vi "Init_UI_Cluster.vi"(0 "UI_Cluster_In":T1, 3 "error in":errorcluster) -> (7 "UI_Cluster_Out":T1, 10 "error out":errorcluster)   [LabVIEW 2020]
uses:
  Type_Def/UI_Ref_Cluster.ctl
  controls/Car_wash_indicators.ctl
  controls/Wash_options.ctl
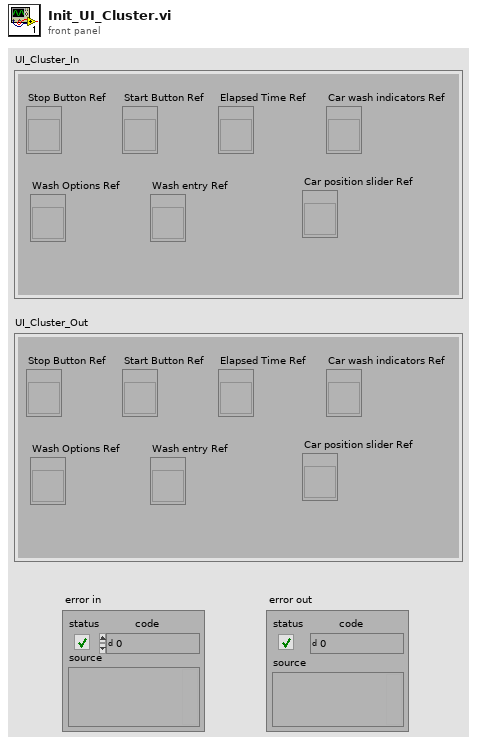
[diagram p1: front panel]
types:
  T1 = typedef "UI_Ref_Cluster.ctl" = cluster{"Stop Button Ref":refnum<vi>, "Start Button Ref":refnum<vi>, "Elapsed Time Ref":refnum<vi>, "Car wash indicators Ref":refnum<vi>, "Wash Options Ref":refnum<vi>, "Wash entry Ref":refnum<vi>, "Car position slider Ref":refnum<vi>}
  T2 = enum8{"Enabled", "Disabled", "Disabled and Grayed Out"}
  T3 = typedef "Wash_options.ctl" = cluster{"Under body wash":bool, "Bug remover":bool, "Pre-soak":bool, "High pressure":bool, "Low pressure":bool, "Spot free Rinse":bool, "Tire Shine Foam":bool, "Air Dry":bool}
  T4 = typedef "Car_wash_indicators.ctl" = cluster{"Under Body Wash":bool, "Bug remover":bool, "Pre-soak":bool, "High pressure Wash":bool, "Low pressure Wax":bool, "Spot free Rinse ":bool, "Tire Shine Foam ":bool, "Air Dry ":bool, "Vehicle Out of Position":bool}
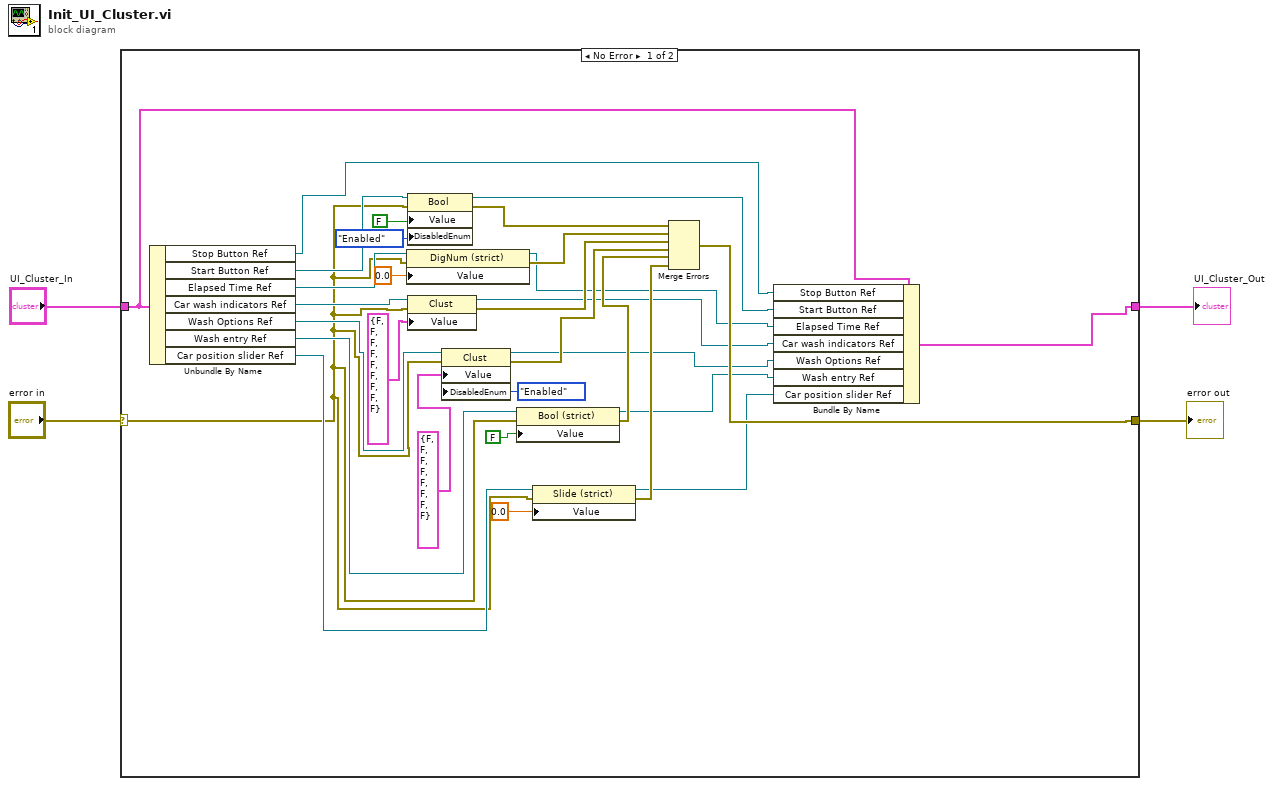
[diagram p0: block diagram]
diagram:
  n1 = case shown="No Error" "error in" {
    selector: "error in" -> [w18 w37]
    tunnel: [w16 w37] -> w3
    tunnel: "UI_Cluster_In" -> [w15 w36]
    tunnel: [w8 w36] -> w1
    frame No Error {
      n2 = Unbundle By Name(w15) -> ("Stop Button Ref"=w7:refnum<vi>, "Start Button Ref"=w35:refnum<vi>, "Elapsed Time Ref"=w32:refnum<vi>, "Car wash indicators Ref"=w29:refnum<vi>, "Wash Options Ref"=w26:refnum<vi>, "Wash entry Ref"=w23:refnum<vi>, "Car position slider Ref"=w22:refnum<vi>)
      n3 = property class="DigNum (strict)"(reference=w32, error in=w18, "Value"=0.0) -> (reference out=w13:refnum<vi>, error out=w30:errorcluster)
      n4 = property class="Bool"(reference=w35, error in=w18, "Value"=FALSE, "DisabledEnum"=T2."Enabled" ("Disabled")) -> (reference out=w14:refnum<vi>, error out=w33:errorcluster)
      n5 = property class="Clust"(reference=w29, error in=w18, "Value"=T4 {"Under Body Wash"=FALSE, "Bug remover"=FALSE, "Pre-soak"=FALSE, "High pressure Wash"=FALSE, "Low pressure Wax"=FALSE, "Spot free Rinse "=FALSE, "Tire Shine Foam "=FALSE, "Air Dry "=FALSE, "Vehicle Out of Position"=FALSE} ("Car wash indicators")) -> (reference out=w12:refnum<vi>, error out=w28:errorcluster)
      n6 = property class="Clust"(reference=w26, error in=w18, "Value"=T3 {"Under body wash"=FALSE, "Bug remover"=FALSE, "Pre-soak"=FALSE, "High pressure"=FALSE, "Low pressure"=FALSE, "Spot free Rinse"=FALSE, "Tire Shine Foam"=FALSE, "Air Dry"=FALSE} ("Wash Options"), "DisabledEnum"=T2."Enabled" ("Disabled")) -> (reference out=w11:refnum<vi>, error out=w24:errorcluster)
      n7 = property class="Bool (strict)"(reference=w23, error in=w18, "Value"=FALSE) -> (reference out=w10:refnum<vi>, error out=w20:errorcluster)
      n8 = property class="Slide (strict)"(reference=w22, error in=w18, "Value"=0.0) -> (reference out=w9:refnum<vi>, error out=w17:errorcluster)
      n9 = Merge Errors(w33, w30, w28, w24, w20, w17) -> (w16:errorcluster)
      n10 = Bundle By Name(cluster=w15, "Stop Button Ref"=w7, "Start Button Ref"=w14, "Elapsed Time Ref"=w13, "Car wash indicators Ref"=w12, "Wash Options Ref"=w11, "Wash entry Ref"=w10, "Car position slider Ref"=w9) -> (w8:T1)
    }
    frame Error {
    }
  }
  "UI_Cluster_Out" <- w1
  "error out" <- w3
